vi "FindInterfacesInterface.vi"(2 "Interface":T1, 3 "Interfaces":T1[](array[typedef])) -> (0 "Index":i32, 1 "Found":bool)   [LabVIEW 2020]
uses:
  <vilib>/WebServerConfig/Interface.ctl
panel:
  out "error out":errorcluster
  in  "error in (no error)":errorcluster
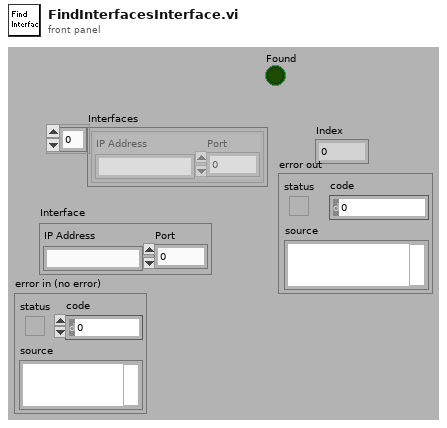
[diagram p1: front panel]
types:
  T1 = typedef "Interface.ctl" = cluster{"IP Address":string, "Port":u16}
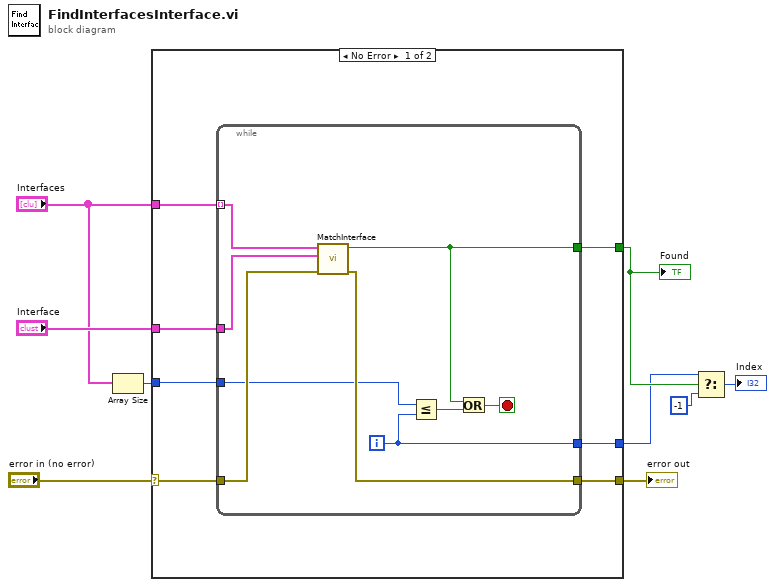
[diagram p0: block diagram]
diagram:
  n1 = Array Size(array="Interfaces") -> (size(s)=w5:i32)
  n2 = case shown="No Error" "error in (no error)" {
    selector: "error in (no error)" -> [w13 w26]
    tunnel: "Interfaces" -> [w16 _]
    tunnel: "Interface" -> [w15 _]
    tunnel: [w14 w26] -> w8
    tunnel: w5 -> [w12 _]
    tunnel: [w11 _] -> w4
    tunnel: [w10 _] -> w3
    frame No Error {
      n3 = while {
        tunnel: [w21] -> w10
        tunnel: w16 -> [w25] mode=indexing
        tunnel: w15 -> [w24]
        tunnel: w13 -> [w23]
        tunnel: [w22] -> w14
        tunnel: w12 -> [w20]
        tunnel: [w17] -> w11
        i -> [w21]
        stop <- w18 stop-if-true
        n4 = call <vilib>:"MatchInterface.vi"("error in (no error)"=w23, "Interface 2"=w24, "Interface 1"=w25) -> ("error out"=w22:errorcluster, "Matches"=w17:bool)  [unwired: 6 in, 1 out]
        n5 = Less Or Equal?(x=w20, y=w21) -> (x <= y?=w19:bool)
        n6 = Or(x=w17, y=w19) -> (x .or. y?=w18:bool)
      }
    }
    frame Error {
    }
  }
  "error out" <- w8
  "Found" <- w4
  n7 = Select(t=w3, s=w4, f=-1) -> (s? t:f=→"Index":i32)
